vi "Determine Rectangle Points.vi"(8 "error in (no error)":errorcluster, 11 "Tool Rectangle in":refnum<class "Tool Rectangle.lvclass">) -> (0 "error out":errorcluster, 2 "interleaved array":cluster{"X":dbl, "Y":dbl}[](array[cluster]), 3 "Tool Rectangle out":refnum<class "Tool Rectangle.lvclass">)   [LabVIEW 2019, in "Tool Rectangle.lvclass"]
uses:
  Tool Rectangle.lvclass
  Settings/Rectangle Settings/Rectangle Settings.lvclass/Rectangle Settings.ctl
  Settings/Rectangle Settings/Accessors/Read Fill Orientation.vi
  Settings/Rectangle Settings/Rectangle Settings.lvclass
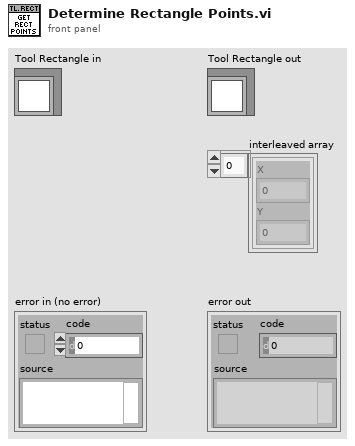
[diagram p1: front panel]
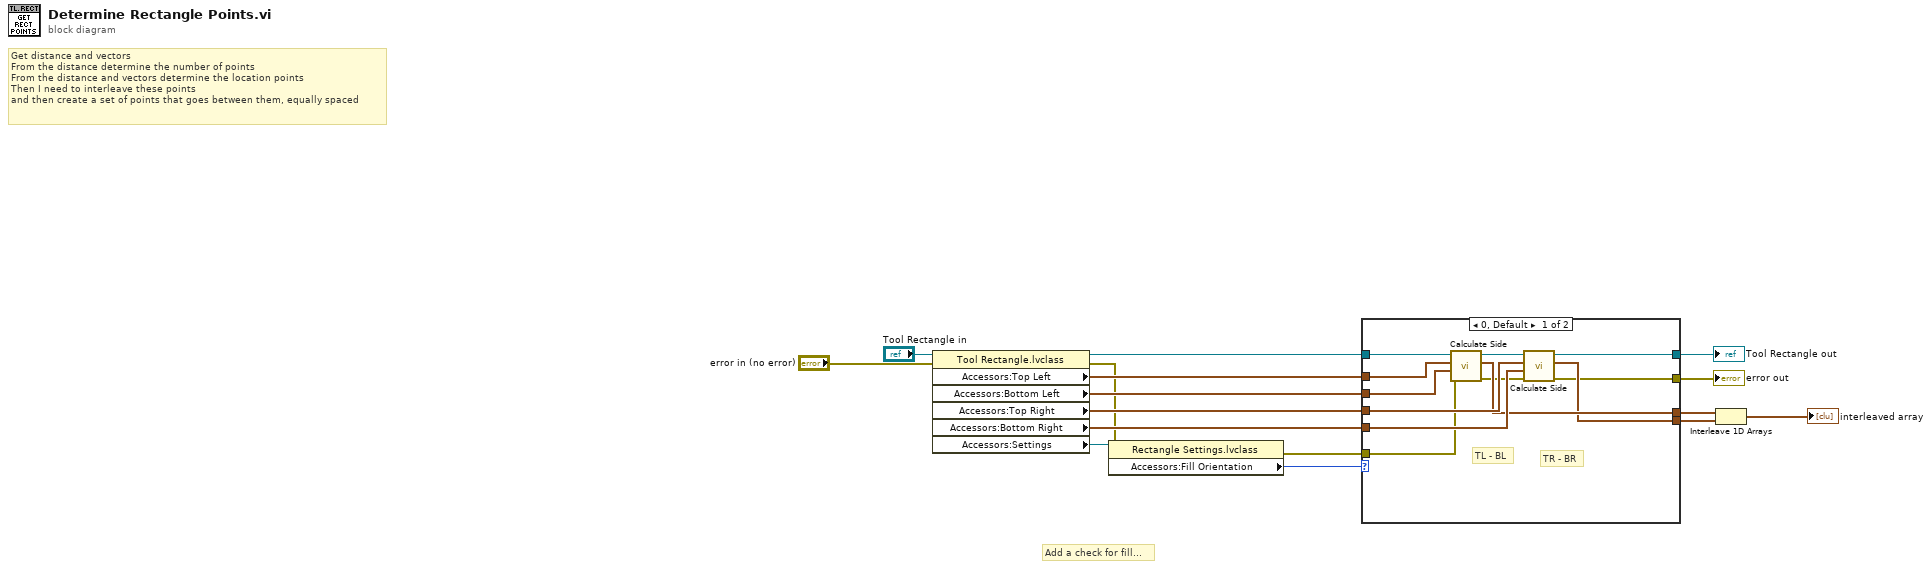
[diagram p0: block diagram]
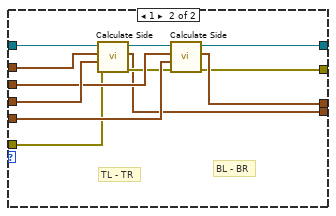
[diagram p2: hidden frame]
diagram:
  # "Add a check for fill..."
  # "Get distance and vectors\nFrom the distance determine the number of points\nFrom the distance and vectors determine the location points\nThen I need to interleave these points\nand then create a set of points that goes between them, equally spaced"
  n1 = property class="Tool Rectangle.lvclass"(reference="Tool Rectangle in", error in="error in (no error)") -> (reference out=w16:refnum<class "Tool Rectangle.lvclass">, error out=w3:errorcluster, "Accessors:Top Left"=w14:cluster{"X":dbl, "Y":dbl}, "Accessors:Bottom Left"=w12:cluster{"X":dbl, "Y":dbl}, "Accessors:Top Right"=w13:cluster{"X":dbl, "Y":dbl}, "Accessors:Bottom Right"=w10:cluster{"X":dbl, "Y":dbl}, "Accessors:Settings"=w11:refnum<class "Rectangle Settings.lvclass">)
  n2 = property class="Rectangle Settings.lvclass"(reference=w11, error in=w3) -> (error out=w2:errorcluster, "Accessors:Fill Orientation"=w6:u16)  [unwired: 1 out]
  n3 = case shown="0, Default" w6 {
    tunnel: [w24 w37] -> w15
    tunnel: w16 -> [w28 w40]
    tunnel: w14 -> [w27 w39]
    tunnel: w12 -> [w26 w35]
    tunnel: w13 -> [w23 w36]
    tunnel: w10 -> [w22 w34]
    tunnel: [w21 w32] -> w9
    tunnel: [w20 w31] -> w8
    tunnel: [w19 w29] -> w4
    tunnel: w2 -> [w18 w30]
    frame 0, Default {
      # "TR - BR"
      # "TL - BL"
      n4 = call-dynamic "Calculate Side.vi"("error in (no error)"=w18, "Point 2"=w26, "Point 1"=w27, "Tool Rectangle in"=w28) -> ("error out"=w17:errorcluster, "Array"=w21:cluster{"X":dbl, "Y":dbl}[], "Tool Rectangle out"=w25:refnum<class "Tool Rectangle.lvclass">)  [unwired: 5 in]
      n5 = call-dynamic "Calculate Side.vi"("error in (no error)"=w17, "Point 2"=w22, "Point 1"=w23, "Tool Rectangle in"=w25) -> ("error out"=w19:errorcluster, "Array"=w20:cluster{"X":dbl, "Y":dbl}[], "Tool Rectangle out"=w24:refnum<class "Tool Rectangle.lvclass">)  [unwired: 5 in]
    }
    frame 1 {
      # "BL - BR"
      # "TL - TR"
      n6 = call-dynamic "Calculate Side.vi"("error in (no error)"=w30, "Point 2"=w36, "Point 1"=w39, "Tool Rectangle in"=w40) -> ("error out"=w33:errorcluster, "Array"=w31:cluster{"X":dbl, "Y":dbl}[], "Tool Rectangle out"=w38:refnum<class "Tool Rectangle.lvclass">)  [unwired: 5 in]
      n7 = call-dynamic "Calculate Side.vi"("error in (no error)"=w33, "Point 2"=w34, "Point 1"=w35, "Tool Rectangle in"=w38) -> ("error out"=w29:errorcluster, "Array"=w32:cluster{"X":dbl, "Y":dbl}[], "Tool Rectangle out"=w37:refnum<class "Tool Rectangle.lvclass">)  [unwired: 5 in]
    }
  }
  "error out" <- w4
  "Tool Rectangle out" <- w15
  n8 = Interleave 1D Arrays(w9, w8) -> (→"interleaved array":cluster{"X":dbl, "Y":dbl}[])
